vi "Real Time Display.vi"() -> ()   [LabVIEW 2015]
uses:
  Type/_Run Mode.ctl
  InternalTools/IonicsServiceTool/Print.ctl
  Type/_Data Operation.ctl
  Type/_RT Command.ctl
  Configuration/_Global Configuration.vi
  <vilib>/Utility/config.llb/Read Key (String).vi
  <vilib>/Utility/config.llb/Read Key (Double).vi
  <vilib>/Utility/config.llb/Read Key (I32).vi
  <vilib>/Utility/NIReport.llb/Append Image to Report (path wrap).vi
  <vilib>/Utility/NIReport.llb/NI_report.lvclass
  <vilib>/Utility/config.llb/NI_LVConfig.lvlib
panel:
  out "Close":bool
  out "Quit":bool=TRUE
  out "Q2DC POL":bool
  out "Q1DC POL":bool
  out "Date":string
  out "MCA":bool
  out "Run Mode":T1
  out "Q2 Resolution":i32[](listbox) caption="Q2 +ve High Res"
  out "Q1 Resolution":i32[](listbox) caption="Q1 +ve High Res"
  out "Q2 Calibration":i32[](listbox)
  out "Q1 Calibration":i32[](listbox)
  out "Scan #":i32=1
  out "Peak List":i32[](listbox)
  out "Lens Values":i32[](listbox)
  out "TIC":cluster{"TIC X":dbl[], "TIC Y":dbl[]}[](graph)
  out "Run Time":i32=1 caption="Run Time (ms)"
  in  "Expt#":i32=1 caption="Experiment #"
  out "Init":bool
  out "A 6":bool
  out "A 5":bool
  out "A 4":bool
  out "A 3":bool
  out "A 2":bool
  out "A 1":bool
  out "MR 5":cluster{dbl[], dbl[]}(graph)
  out "MR 4":cluster{dbl[], dbl[]}(graph)
  out "MR 2":cluster{dbl[], dbl[]}(graph)
  out "MR 1":cluster{dbl[], dbl[]}(graph)
  out "MR 6":cluster{dbl[], dbl[]}(graph)
  out "MR 3":cluster{dbl[], dbl[]}(graph)
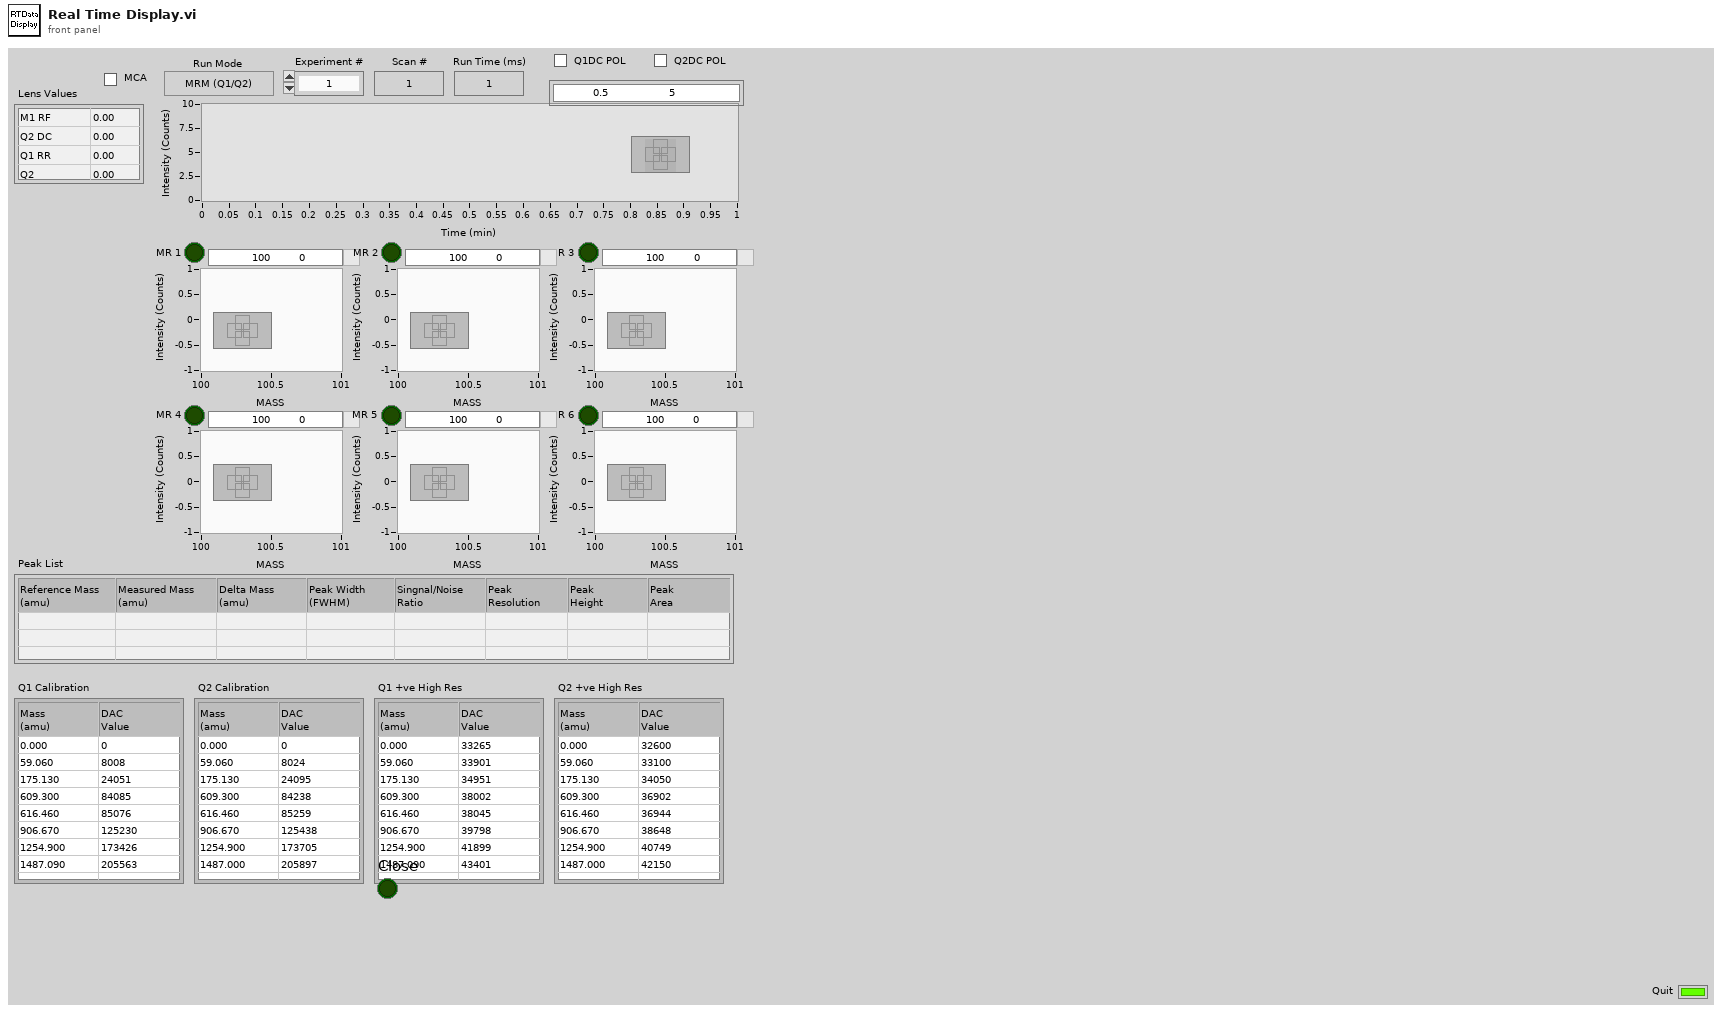
[diagram p1: front panel]
types:
  T1 = typedef "_Run Mode.ctl" = enum16{"MRM (Q1/Q2)", "Q1 Scan", "Q1 SRM", "Q2 Scan", "Q2 SRM", "Product Scan", "Precursor Scan", "Neutral Loss", "Neutral Gain"}
  T2 = cluster{"TIC":refnum<vi>, "MR 1":refnum<vi>, "MR 2":refnum<vi>, "MR 3":refnum<vi>, "MR 4":refnum<vi>, "MR 5":refnum<vi>, "MR 6":refnum<vi>, "A 1":refnum<vi>, "A 2":refnum<vi>, "A 3":refnum<vi>, "A 4":refnum<vi>, "A 5":refnum<vi>, "A 6":refnum<vi>, "Lens Values":refnum<vi>, "Q1 Calibration":refnum<vi>, "Q2 Calibration":refnum<vi>, "Q1 Resolution":refnum<vi>, "Q2 Resolution":refnum<vi>, "Peak List":refnum<vi>}
  T3 = cluster{"RefMass":dbl[], "LensList":i32[], "SearchWin":dbl, "MinH":dbl, "MinW":i32, "RunTime":i32}
  T4 = typedef "Print.ctl" = cluster{"Picture Name":string, "VI Reference":refnum<vi>}
  T5 = enum16{"Standard Report", "HTML", "Word", "Excel"}
  T6 = typedef "_Data Operation.ctl" = enum8{"Initialize", "Get Data", "Set Data", "Close"}
  T7 = typedef "_RT Command.ctl" = enum16{"xml Start Run", "xml Start Actual Run", "xml Stop Run", "xml Runtime Update", "xml Get Status", "xml Get Table", "xml Set Table", "xml Get Configuration", "xml System Status", "xml Set LC Input Logic", "xml Get Data", "xml Get Info", "Start", "StartActualRun", "Stop", "Runtime Update", "Get Data", "Get Info", "Get Status", "Get Param", "Get Config", "Get Table", "Read ADC", "Set Oscillator", "Update Config", "Update Table", "Set All Pol", "Set Pol and DC", "Set Max Mass", "Toggle RP", "Toggle EL", "Set PIC", "Initialize Turbo", "Send Turbo Comm", "Close Turbo", "P1", "P2", "P3", "Send Serial", "Set LC Out", "Get LC In", "Read VAC", "Test Table", "Toggle Power", "Get Startup", "Set Startup", "Get ADC Table", "Set ADC Table", "Get Brief Status", "Get Detail Status", "Auxiliary Update", "Set CC Logics", "Set CC Input Logics", "Ignore Error", "invalid"}
  T8 = typedef "NI_LVConfig.lvlib/Config Data RefNum.ctl" = refnum<k1>
  T9 = typedef "_Current Data.ctl" = cluster{"Scan#":i32, "Run Time (mS)":i32, "TIC X":dbl[], "TIC Y":dbl[][], "MassRange":cluster{"X Title":string, "X":dbl[], "Y":i32[]}[], "Fixed Mass (amu)":dbl, "Method":T10}
  T10 = typedef "_XML Expt.ctl" = cluster{"StartT(mS)":i32, "#Cycles":i32, "PauseT(uS)":i32, "ScanType":i32, "Polarity":u8, "FixedMass":dbl, "DelayT(mS)":i32, "Active Ch":T11[], "Mass Range":T12[]}
  T11 = typedef "_XML Lens.ctl" = cluster{"Value":dbl, "ChID":u8}
  T12 = typedef "_Mass Range Property.ctl" = cluster{"Start":dbl, "Stop":dbl, "Step Size":dbl, "Steps":i32, "Dwell":dbl, "Parameters":T13[], "Res":T14}
  T13 = typedef "_Mass Range Parameters.ctl" = cluster{"Name":string, "Ch#":u8, "StartV":dbl, "StopV":dbl, "StepV":dbl, "Index":u8}
  T14 = typedef "_RT Res Type.ctl" = u16
  T15 = typedef "_Peak Property.ctl" = cluster{"Centroid":dbl, "Height":dbl, "FWHM":dbl, "Resolution":dbl, "Area":dbl, "StoN":dbl, "ApexX":dbl, "Baseline":dbl, "LEdgeX":dbl, "LEdgeY":dbl, "REdgeX":dbl, "REdgeY":dbl, "LEdgeFWHM":dbl, "REdgeFWHM":dbl}
  T16 = typedef "imagedata.ctl" = cluster{"image type":i32, "image depth":i32, "image":u8[], "mask":u8[], "colors":u32[], "Rectangle":cluster{"left":i16, "top":i16, "right":i16, "bottom":i16}}
  T17 = typedef "LVRangeTypeDef.ctl" = cluster{"Minimum":dbl, "Maximum":dbl, "Increment":dbl, "Minor Increment":dbl, "Start":dbl}
  T18 = typedef "LVPointDoubleTypeDef.ctl" = cluster{"Cursor X":dbl, "Cursor Y":dbl}
  T19 = cluster{"YScale.NameLbl.Text":string, "XScale.NameLbl.Text":string, "XScale.Range":T17, "YScale.Range":T17, "Label.Text":string, "Cursor.Cursor Position":T18, "Plot.Bar Plot Style":u8}
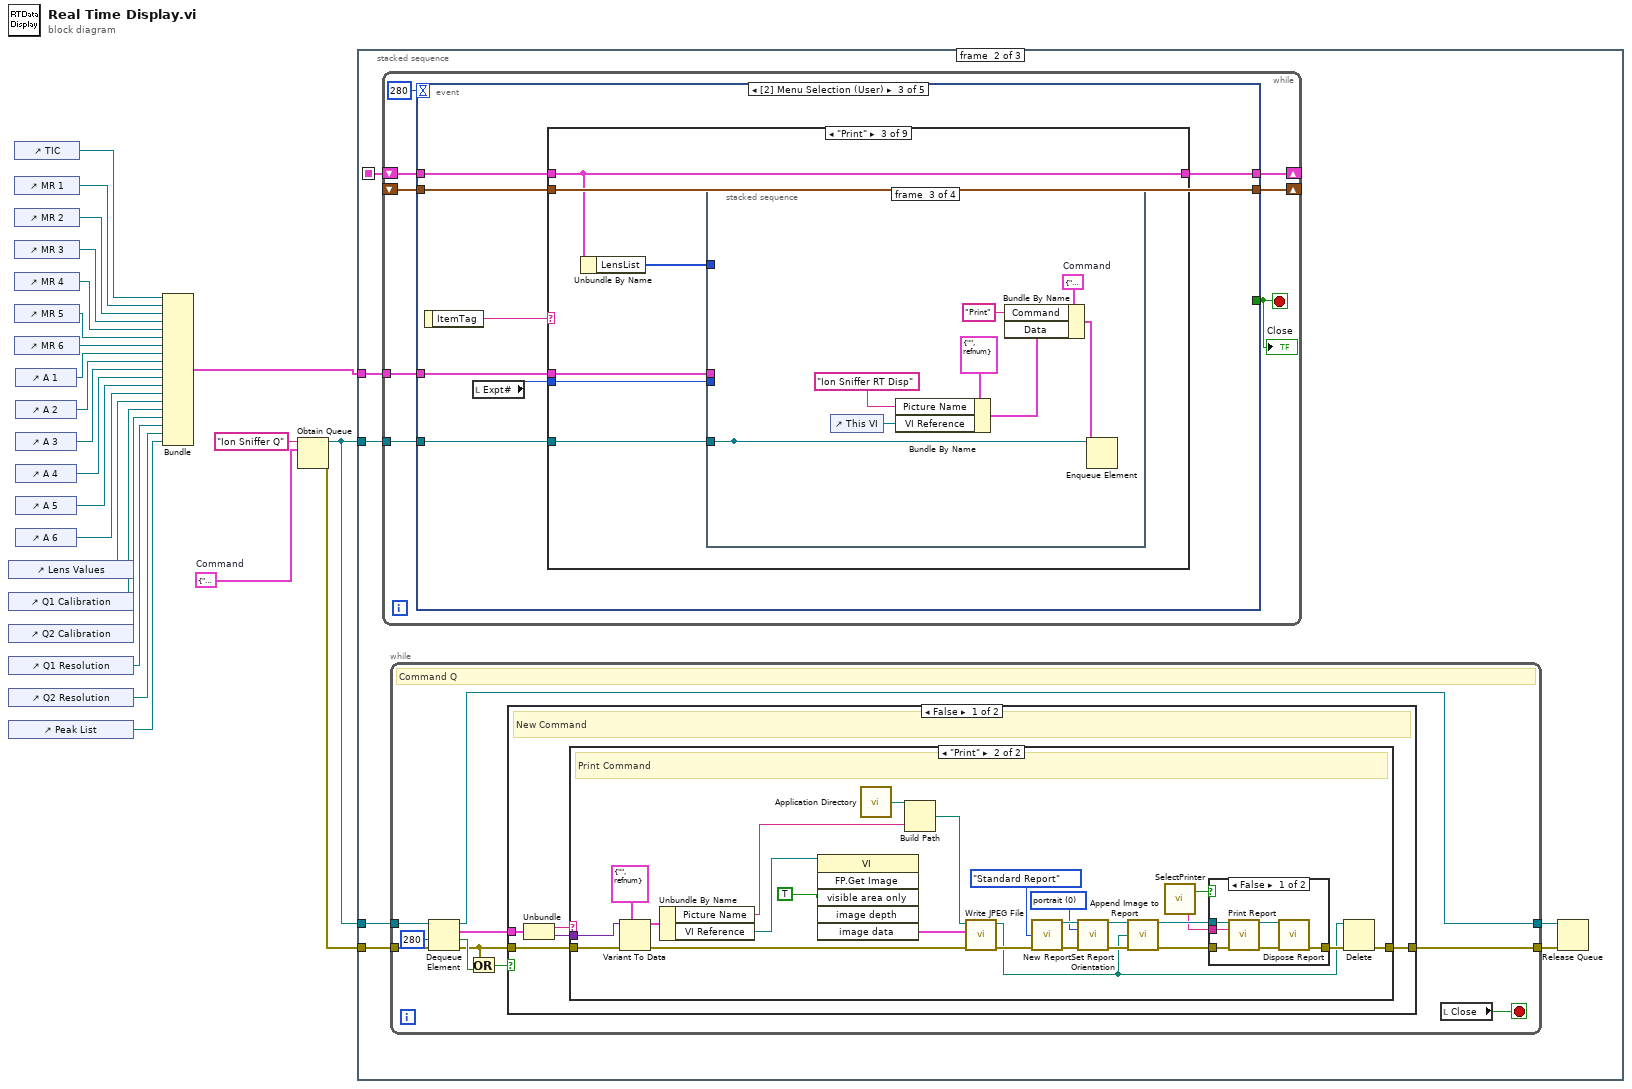
[diagram p0: block diagram]
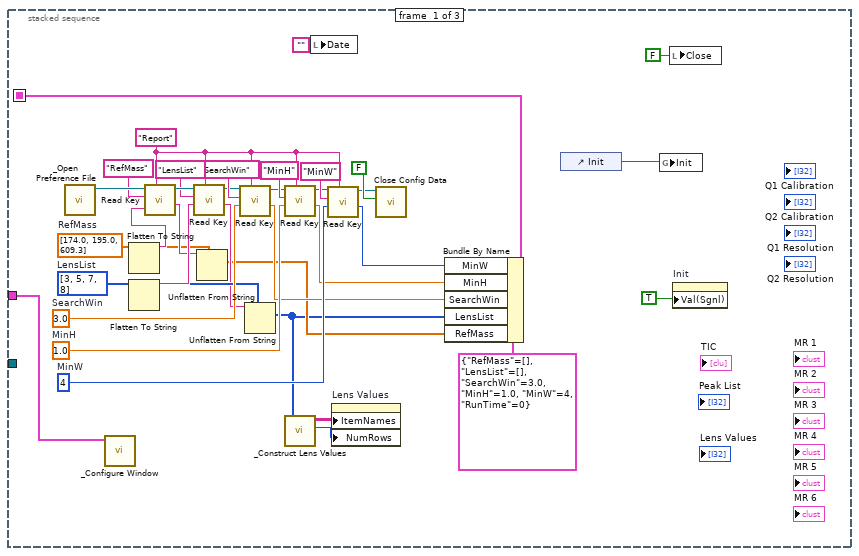
[diagram p2: hidden frame]
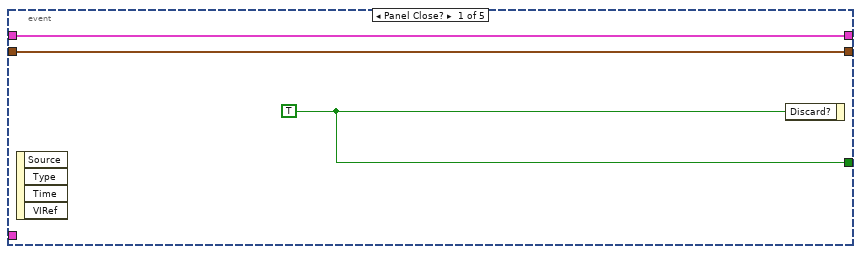
[diagram p6: hidden frame]
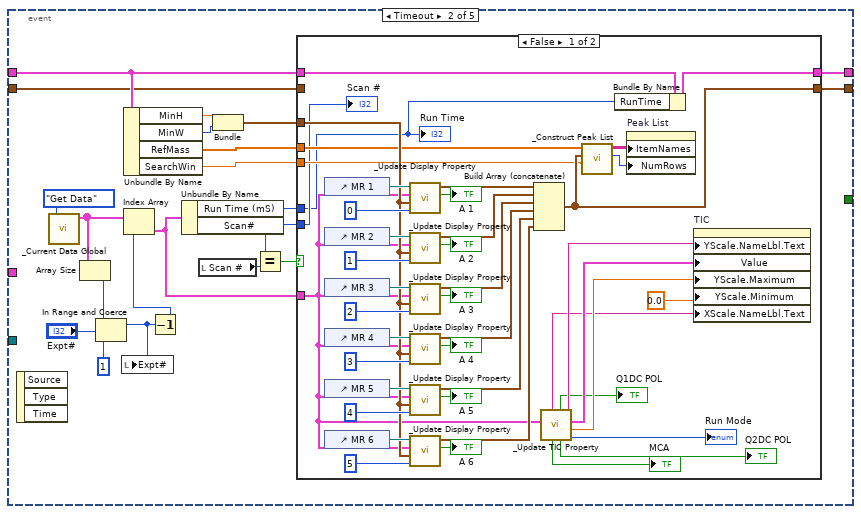
[diagram p7: hidden frame]
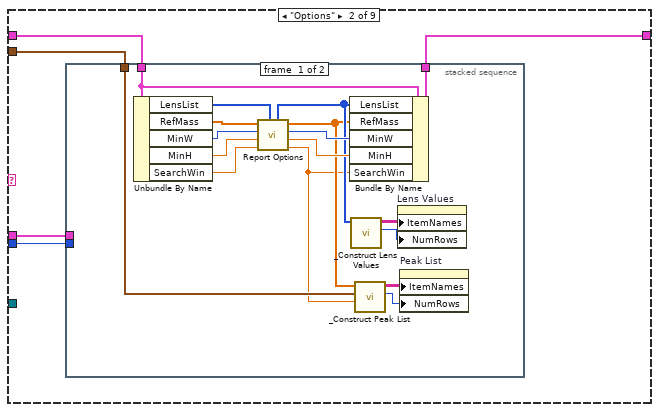
[diagram p10: hidden frame]
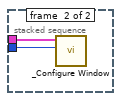
[diagram p11: hidden frame]
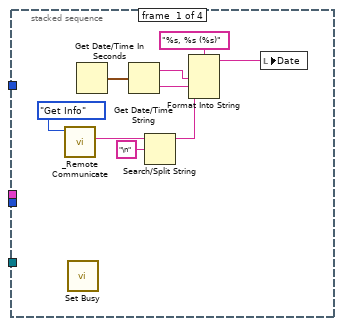
[diagram p12: hidden frame]
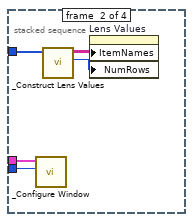
[diagram p13: hidden frame]
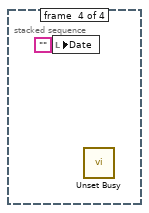
[diagram p14: hidden frame]
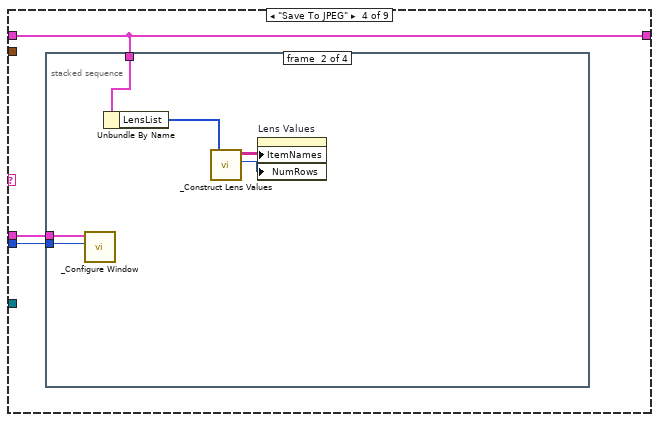
[diagram p15: hidden frame]
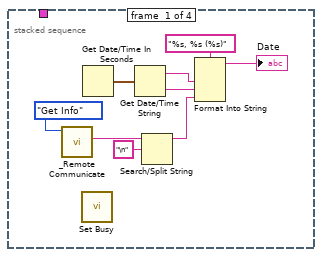
[diagram p16: hidden frame]
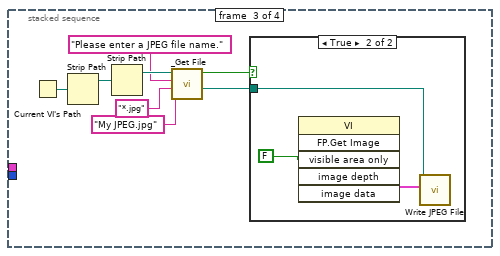
[diagram p17: hidden frame]
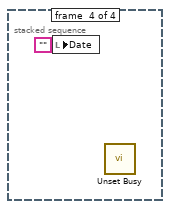
[diagram p19: hidden frame]
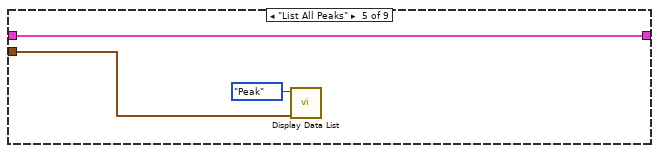
[diagram p20: hidden frame]
diagram:
  w1 = cluster{"Command":string, "Data":variant} {"Command"="", "Data"=variant}  # Command
  n1 = control-ref of="Lens Values"() -> (w24:refnum<vi>)
  n2 = control-ref of="Q1 Calibration"() -> (w10:refnum<vi>)
  n3 = control-ref of="Q2 Calibration"() -> (w9:refnum<vi>)
  n4 = control-ref of="Q1 Resolution"() -> (w8:refnum<vi>)
  n5 = control-ref of="Q2 Resolution"() -> (w7:refnum<vi>)
  n6 = control-ref of="Peak List"() -> (w6:refnum<vi>)
  n7 = control-ref of="TIC"() -> (w5:refnum<vi>)
  n8 = control-ref of="MR 1"() -> (w12:refnum<vi>)
  n9 = control-ref of="MR 2"() -> (w13:refnum<vi>)
  n10 = control-ref of="MR 3"() -> (w14:refnum<vi>)
  n11 = control-ref of="MR 4"() -> (w15:refnum<vi>)
  n12 = control-ref of="MR 5"() -> (w16:refnum<vi>)
  n13 = control-ref of="MR 6"() -> (w17:refnum<vi>)
  n14 = control-ref of="A 1"() -> (w18:refnum<vi>)
  n15 = control-ref of="A 2"() -> (w19:refnum<vi>)
  n16 = control-ref of="A 3"() -> (w20:refnum<vi>)
  n17 = control-ref of="A 4"() -> (w21:refnum<vi>)
  n18 = control-ref of="A 5"() -> (w22:refnum<vi>)
  n19 = control-ref of="A 6"() -> (w23:refnum<vi>)
  n20 = Bundle("TIC"=w5, "MR 1"=w12, "MR 2"=w13, "MR 3"=w14, "MR 4"=w15, "MR 5"=w16, "MR 6"=w17, "A 1"=w18, "A 2"=w19, "A 3"=w20, "A 4"=w21, "A 5"=w22, "A 6"=w23, "Lens Values"=w24, "Q1 Calibration"=w10, "Q2 Calibration"=w9, "Q1 Resolution"=w8, "Q2 Resolution"=w7, "Peak List"=w6) -> (w11:T2)  [unwired: 1 out]
  n21 = Obtain Queue(name (unnamed)="Ion Sniffer Q", element data type=w1) -> (queue out=w3:refnum<queue>, error out=w2:errorcluster)  [unwired: 3 in, 1 out]
  n22 = stacked-sequence {
    seq-local: [w31 _ _] -> [_ w67 _]
    tunnel: w11 -> [w27 w66 _]
    tunnel: w3 -> [_ w65 _]
    tunnel: w3 -> [_ w64 _]
    tunnel: w2 -> [_ w63 _]
    frame #0 {
      w47 = "Report" ("section")
      w38 = i32[] [3, 5, 7, 8]  # LensList
      w43 = 4  # MinW
      w44 = 1.0  # MinH
      w45 = 3.0  # SearchWin
      w39 = dbl[] [174.0, 195.0, 609.3]  # RefMass
      n23 = call "_Open Preference File.vi"() -> ("refnum"=w56:T8)  [unwired: 3 in, 4 out]
      n24 = call "_Configure Window.vi"("ControlRef"=w27) -> ()  [unwired: 2 in, 5 out]
      n25 = Flatten To String(anything=w39) -> (data string=w42:string)  [unwired: 1 in, 4 out]
      n26 = Flatten To String(anything=w38) -> (data string=w41:string)  [unwired: 1 in, 4 out]
      n27 = call-poly <vilib>:"Read Key.vi"("section"=w47, "default value"=w42, "key"="RefMass", "refnum"=w56) -> ("value"=w40:string, "refnum out"=w58:T8)  [unwired: 2 in, 4 out]
      n28 = call-poly <vilib>:"Read Key.vi"("section"=w47, "default value"=w41, "key"="LensList" ("section"), "refnum"=w58) -> ("value"=w37:string, "refnum out"=w50:T8)  [unwired: 2 in, 4 out]
      n29 = Unflatten From String(type=w39, binary string=w40) -> (value=w32:dbl[])  [unwired: 1 in, 4 out]
      n30 = call-poly <vilib>:"Read Key.vi"("section"=w47, "default value"=w45, "key"="SearchWin", "refnum"=w50) -> ("value"=w33:dbl, "refnum out"=w51:T8)  [unwired: 1 in, 5 out]
      n31 = Unflatten From String(type=w38, binary string=w37) -> (value=w30:i32[])  [unwired: 1 in, 4 out]
      n32 = call-poly <vilib>:"Read Key.vi"("section"=w47, "default value"=w44, "key"="MinH" ("section"), "refnum"=w51) -> ("value"=w34:dbl, "refnum out"=w48:T8)  [unwired: 1 in, 5 out]
      n33 = call "_Construct Lens Values.vi"("Lens List"=w30) -> ("# of Lens"=w28:i32, "Table"=w29:string[][])  [unwired: 5 out]
      n34 = local write "Date"("") -> ()
      n35 = call-poly <vilib>:"Read Key.vi"("section"=w47, "default value"=w43, "key"="MinW" ("section"), "refnum"=w48) -> ("value"=w35:i32, "refnum out"=w46:T8)  [unwired: 1 in, 5 out]
      n36 = property on="Lens Values" class="MCListbox (strict)"("ItemNames"=w29, "NumRows"=w28) -> ()  [unwired: 2 in, 2 out]
      n37 = call <vilib>:"Close Config Data.vi"("write file if changed (T)"=FALSE ("write configuration file? (F)"), "refnum"=w46) -> ()  [unwired: 1 in, 9 out]
      n38 = Bundle By Name(cluster=T3 {"RefMass"=[], "LensList"=[], "SearchWin"=3.0, "MinH"=1.0, "MinW"=4, "RunTime"=0}, "MinW"=w35, "MinH"=w34, "SearchWin"=w33, "LensList"=w30, "RefMass"=w32) -> (w31:T3)
      n39 = control-ref of="Init"() -> (w60:refnum<vi>)
      n40 = global write "_Global Configuration.vi" "Init"(w60) -> ()
      n41 = local write "Close"(FALSE ("Close")) -> ()
      n42 = property on="Init" class="Bool (strict)"("Val(Sgnl)"=TRUE ("Value (Signaling)")) -> ()  [unwired: 2 in, 2 out]
    }
    frame #1 {
      n43 = while {
        shift-right: [w123] -> _
        shift-left: w67 -> [w124]
        shift-right: [w122] -> _
        shift-left: _ -> [w121]
        tunnel: w66 -> [w120]
        tunnel: w65 -> [w118]
        stop <- w117 stop-if-true
        n44 = event shown="[2] Menu Selection (User)" {
          selector: _ -> [_ _ _ _ _]
          dyn-events: _ -> [_ _ _ _ _]
          timeout: 280 -> [_ _ _ _ _]
          tunnel: [w127 _ _ _ _] -> w117
          tunnel: w124 -> [w126 w148 w200 w312 w318]
          tunnel: [w126 w147 w199 w313 w318] -> w123
          tunnel: [w125 w145 w198 w308 w317] -> w122
          tunnel: w121 -> [w125 w146 w198 w308 w317]
          tunnel: w120 -> [_ _ w197 w306 _]
          tunnel: w118 -> [_ _ w195 _ _]
          event Panel Close? {
            w127 = TRUE ("Discard?")
            n45 = event-data() -> ()  [unwired: 5 out]
            n46 = event-data("Discard?"=w127) -> ()  [unwired: 1 in, 1 out]
          }
          event Timeout {
            n47 = event-data() -> ()  [unwired: 4 out]
            n48 = call "_Current Data Global.vi"("Operation"=_Data_Operation."Get Data") -> ("CurrentData"=w137:T9[])  [unwired: 3 in, 3 out]
            n49 = Array Size(array=w137) -> (size(s)=w134:i32)
            n50 = In Range and Coerce(upper limit=w134, x="Expt#", lower limit=1) -> (coerced(x)=w133:i32)  [unwired: 1 out]
            n51 = local write "Expt#"(w133) -> ()
            n52 = Unbundle By Name(w148) -> ("MinH"=w143:dbl, "MinW"=w142:i32, "RefMass"=w140:dbl[], "SearchWin"=w139:dbl)
            n53 = Decrement(x=w133) -> (x-1=w132:i32)
            n54 = Index Array(array=w137, index=w132) -> (element=w138:T9)
            n55 = Unbundle By Name(w138) -> ("Run Time (mS)"=w128:i32, "Scan#"=w130:i32)
            n56 = local read "Scan #"() -> (w131:i32)
            n57 = Bundle("MinH"=w143, "MinW"=w142) -> (w141:cluster{"MinH":dbl, "MinW":i32})  [unwired: 1 out]
            n58 = Equal?(x=w130, y=w131) -> (x = y?=w129:bool)
            n59 = case shown="False" w129 {
              tunnel: w148 -> [w192 w194]
              tunnel: [w191 w194] -> w147
              tunnel: [w163 w193] -> w145
              tunnel: w146 -> [_ w193]
              tunnel: w141 -> [w177 _]
              tunnel: w138 -> [w159 _]
              tunnel: w140 -> [w162 _]
              tunnel: w139 -> [w161 _]
              tunnel: w130 -> [w160 _]
              tunnel: w128 -> [w152 _]
              frame False {
                n60 = control-ref of="MR 1"() -> (w190:refnum<vi>)
                n61 = control-ref of="MR 2"() -> (w189:refnum<vi>)
                n62 = control-ref of="MR 3"() -> (w187:refnum<vi>)
                n63 = control-ref of="MR 4"() -> (w185:refnum<vi>)
                n64 = control-ref of="MR 5"() -> (w183:refnum<vi>)
                n65 = control-ref of="MR 6"() -> (w181:refnum<vi>)
                n66 = call "_Update Display Property.vi"("MassRange# (0)"=0, "PeakParam"=w177, "Current Data"=w159, "Display Refnum"=w190) -> ("Active"=→"A 1":bool, "Peak List"=w171:T15[])  [unwired: 3 out]
                n67 = call "_Update Display Property.vi"("MassRange# (0)"=1, "PeakParam"=w177, "Current Data"=w159, "Display Refnum"=w189) -> ("Active"=→"A 2":bool, "Peak List"=w170:T15[])  [unwired: 3 out]
                n68 = call "_Update Display Property.vi"("MassRange# (0)"=2, "PeakParam"=w177, "Current Data"=w159, "Display Refnum"=w187) -> ("Active"=→"A 3":bool, "Peak List"=w169:T15[])  [unwired: 3 out]
                n69 = call "_Update Display Property.vi"("MassRange# (0)"=3, "PeakParam"=w177, "Current Data"=w159, "Display Refnum"=w185) -> ("Active"=→"A 4":bool, "Peak List"=w168:T15[])  [unwired: 3 out]
                n70 = call "_Update Display Property.vi"("MassRange# (0)"=4, "PeakParam"=w177, "Current Data"=w159, "Display Refnum"=w183) -> ("Active"=→"A 5":bool, "Peak List"=w167:T15[])  [unwired: 3 out]
                n71 = call "_Update Display Property.vi"("MassRange# (0)"=5, "PeakParam"=w177, "Current Data"=w159, "Display Refnum"=w181) -> ("Active"=→"A 6":bool, "Peak List"=w166:T15[])  [unwired: 3 out]
                n72 = Build Array (concatenate)(w171, w170, w169, w168, w167, w166) -> (w163:T15[])
                n73 = call "_Update TIC Property.vi"("Current Data"=w159) -> ("Run Mode"=→"Run Mode":T1, "YMax"=w156:dbl, "TIC Data"=w157:cluster{"TIC X":dbl[], "Data in cps":dbl[]}[], "YTitle"=w158:string, "Q2DC Pol"=→"Q2DC POL":bool, "Q1DC Pol"=→"Q1DC POL":bool, "MCA"=→"MCA":bool, "XTitle"=w151:string)  [unwired: 3 out]
                n74 = call "_Construct Peak List.vi"("Search Window"=w161, "Peak List"=w163, "RefMass"=w162) -> ("# of Peaks"=w164:i32, "Table"=w165:string[][])  [unwired: 3 out]
                n75 = Bundle By Name(cluster=w192, "RunTime"=w152) -> (w191:T3)
                n76 = property on="Peak List" class="MCListbox (strict)"("ItemNames"=w165, "NumRows"=w164) -> ()  [unwired: 2 in, 2 out]
                n77 = property on="TIC" class="XYGraph (strict)"("YScale.NameLbl.Text"=w158, "Value"=w157, "YScale.Maximum"=w156, "YScale.Minimum"=0.0 ("Y Scale.Range:Minimum"), "XScale.NameLbl.Text"=w151) -> ()  [unwired: 2 in, 2 out]
                "Run Time" <- w152
                "Scan #" <- w160
              }
              frame True {
              }
            }
          }
          event Menu Selection (User) {
            n78 = event-data() -> ("ItemTag"=w201:string)  [unwired: 1 out]
            n79 = local read "Expt#"() -> (w196:i32)
            n80 = case shown="\"Print\"" w201 {
              tunnel: w200 -> [w202 w207 w231 w257 w287 w288 w291 w293 w305]
              tunnel: [w202 w206 w231 w257 w287 w288 w291 w293 w305] -> w199
              tunnel: w198 -> [_ w205 _ _ w286 _ _ _ _]
              tunnel: w197 -> [_ w204 w229 w256 _ _ _ w294 w304]
              tunnel: w196 -> [_ w203 w228 w255 _ _ _ w292 w303]
              tunnel: w195 -> [_ _ w227 _ _ _ _ _ _]
              frame Default {
              }
              frame "Options" {
                n81 = stacked-sequence {
                  tunnel: w207 -> [w208 _]
                  tunnel: [w219 _] -> w206
                  tunnel: w205 -> [w216 _]
                  tunnel: w204 -> [_ w226]
                  tunnel: w203 -> [_ w225]
                  frame #0 {
                    n82 = Unbundle By Name(w208) -> ("LensList"=w224:i32[], "RefMass"=w215:dbl[], "MinW"=w223:i32, "MinH"=w222:dbl, "SearchWin"=w214:dbl)
                    n83 = call "Report Options.vi"("LensList"=w224, "Search Window"=w214, "Min. Height"=w222, "Min. Width"=w223, "RefMass"=w215) -> ("Search Window 2"=w209:dbl, "Min. Height 2"=w220:dbl, "Min. Width 2"=w221:i32, "RefMass 2"=w210:dbl[], "LensList 2"=w211:i32[])
                    n84 = Bundle By Name(cluster=w208, "LensList"=w211, "RefMass"=w210, "MinW"=w221, "MinH"=w220, "SearchWin"=w209) -> (w219:T3)
                    n85 = call "_Construct Lens Values.vi"("Lens List"=w211) -> ("# of Lens"=w212:i32, "Table"=w213:string[][])  [unwired: 5 out]
                    n86 = call "_Construct Peak List.vi"("Search Window"=w209, "Peak List"=w216, "RefMass"=w210) -> ("# of Peaks"=w217:i32, "Table"=w218:string[][])  [unwired: 3 out]
                    n87 = property on="Lens Values" class="MCListbox (strict)"("ItemNames"=w213, "NumRows"=w212) -> ()  [unwired: 2 in, 2 out]
                    n88 = property on="Peak List" class="MCListbox (strict)"("ItemNames"=w218, "NumRows"=w217) -> ()  [unwired: 2 in, 2 out]
                  }
                  frame #1 {
                    n89 = call "_Configure Window.vi"("Expt#"=w225, "ControlRef"=w226) -> ()  [unwired: 1 in, 5 out]
                  }
                }
              }
              frame "Print" {
                n90 = Unbundle By Name(w231) -> ("LensList"=w230:i32[])
                n91 = stacked-sequence {
                  tunnel: w230 -> [_ w243 _ _]
                  tunnel: w229 -> [_ w242 _ _]
                  tunnel: w228 -> [_ w241 _ _]
                  tunnel: [_ _ w253 _] -> _
                  tunnel: w227 -> [_ _ w253 _]
                  frame #0 {
                    n92 = call "_Remote Communicate.vi"("Command"=_RT_Command."Get Info") -> ("Info"=w239:string)  [unwired: 5 in, 3 out]
                    n93 = call <vilib>:"Set Busy.vi"() -> ()  [unwired: 4 in, 8 out]
                    n94 = Get Date/Time In Seconds() -> (seconds since 1Jan1904=w237:timestamp)
                    n95 = Get Date/Time String(seconds (now)=w237) -> (date string=w235:string, time string=w234:string)  [unwired: 2 out]
                    n96 = Search/Split String(string=w239, search string/char (-)="\n") -> (substring before match=w233:string)  [unwired: 3 out]
                    n97 = Format Into String(format string="%s, %s (%s)", w235, w234, w233) -> (resulting string=w232:string)  [unwired: 2 in, 1 out]
                    n98 = local write "Date"(w232) -> ()
                  }
                  frame #1 {
                    n99 = call "_Configure Window.vi"("Expt#"=w241, "ControlRef"=w242) -> ()  [unwired: 1 in, 5 out]
                    n100 = call "_Construct Lens Values.vi"("Lens List"=w243) -> ("# of Lens"=w244:i32, "Table"=w245:string[][])  [unwired: 5 out]
                    n101 = property on="Lens Values" class="MCListbox (strict)"("ItemNames"=w245, "NumRows"=w244) -> ()  [unwired: 2 in, 2 out]
                  }
                  frame #2 {
                    w252 = cluster{"Command":string, "Data":variant} {"Command"="", "Data"=variant}  # Command
                    n102 = control-ref of="This VI"() -> (w247:refnum<vi>)
                    n103 = Bundle By Name(cluster=T4 {"Picture Name"="", "VI Reference"=refnum} ("Cluster"), "Picture Name"="Ion Sniffer RT Disp", "VI Reference"=w247) -> (w246:T4)
                    n104 = Bundle By Name(cluster=w252, "Command"="Print", "Data"=w246) -> (w250:cluster{"Command":string, "Data":variant})
                    n105 = Enqueue Element(queue=w253, element=w250) -> ()  [unwired: 2 in, 3 out]
                  }
                  frame #3 {
                    n106 = local write "Date"("") -> ()
                    n107 = call <vilib>:"Unset Busy.vi"() -> ()  [unwired: 2 in, 10 out]
                  }
                }
              }
              frame "Save To JPEG" {
                n108 = stacked-sequence {
                  tunnel: w257 -> [_ w270 _ _]
                  tunnel: w256 -> [_ w268 _ _]
                  tunnel: w255 -> [_ w267 _ _]
                  frame #0 {
                    n109 = call "_Remote Communicate.vi"("Command"=_RT_Command."Get Info") -> ("Info"=w265:string)  [unwired: 5 in, 3 out]
                    n110 = call <vilib>:"Set Busy.vi"() -> ()  [unwired: 4 in, 8 out]
                    n111 = Get Date/Time In Seconds() -> (seconds since 1Jan1904=w263:timestamp)
                    n112 = Get Date/Time String(seconds (now)=w263) -> (date string=w261:string, time string=w260:string)  [unwired: 2 out]
                    n113 = Search/Split String(string=w265, search string/char (-)="\n") -> (substring before match=w259:string)  [unwired: 3 out]
                    n114 = Format Into String(format string="%s, %s (%s)", w261, w260, w259) -> (resulting string=→"Date":string)  [unwired: 2 in, 1 out]
                  }
                  frame #1 {
                    n115 = call "_Configure Window.vi"("Expt#"=w267, "ControlRef"=w268) -> ()  [unwired: 1 in, 5 out]
                    n116 = Unbundle By Name(w270) -> ("LensList"=w269:i32[])
                    n117 = call "_Construct Lens Values.vi"("Lens List"=w269) -> ("# of Lens"=w271:i32, "Table"=w272:string[][])  [unwired: 5 out]
                    n118 = property on="Lens Values" class="MCListbox (strict)"("ItemNames"=w272, "NumRows"=w271) -> ()  [unwired: 2 in, 2 out]
                  }
                  frame #2 {
                    n119 = Current VI's Path() -> (path=w280:path)
                    n120 = Strip Path(path=w280) -> (stripped path=w279:path)  [unwired: 1 out]
                    n121 = Strip Path(path=w279) -> (stripped path=w278:path)  [unwired: 1 out]
                    n122 = call "_Get File.vi"("default name"="My JPEG.jpg", "extension (isd)"="*.jpg", "prompt"="Please enter a JPEG file name.", "Start Path"=w278) -> ("Seleted File"=w274:path, "Succeeded"=w275:bool)  [unwired: 2 in, 2 out]
                    n123 = case shown="True" w275 {
                      tunnel: w274 -> [_ w281]
                      frame False {
                      }
                      frame True {
                        n124 = invoke class="VI" method="FP.Get Image"("visible area only"=FALSE ("Visible Area Only")) -> ("image data"=w282:T16)  [unwired: 5 in, 5 out]
                        n125 = call <vilib>:"Write JPEG File.vi"("image data"=w282, "path to JPEG file"=w281) -> ()  [unwired: 1 in, 9 out]
                      }
                    }
                  }
                  frame #3 {
                    n126 = local write "Date"("") -> ()
                    n127 = call <vilib>:"Unset Busy.vi"() -> ()  [unwired: 2 in, 10 out]
                  }
                }
              }
              frame "List All Peaks" {
                n128 = call "Display Data List.vi"("Peak List"=w286, "Data Type"=enum16{"TIC", "Spectrum", "Peak"}."Peak") -> ()  [unwired: 8 out]
              }
              frame "List TIC Data" {
                n129 = call "Display Data List.vi"("Data Type"=enum16{"TIC", "Spectrum", "Peak"}."TIC") -> ()  [unwired: 3 in, 6 out]
              }
              frame "List Spectral Data" {
                n130 = call "Display Data List.vi"("Data Type"=enum16{"TIC", "Spectrum", "Peak"}."Spectrum") -> ()  [unwired: 1 in, 8 out]
              }
              frame "Show Lens Values" {
                n131 = flat-sequence {
                  tunnel: w294 -> [w296]
                  tunnel: w292 -> [w295]
                  tunnel: w293 -> [w298]
                  frame #0 {
                    n132 = call "_Configure Window.vi"("For Printing (T)"=TRUE ("For Printing (F)"), "Expt#"=w295, "ControlRef"=w296) -> ()  [unwired: 5 out]
                  }
                  frame #1 {
                    n133 = Unbundle By Name(w298) -> ("LensList"=w299:i32[])
                    n134 = call "_Construct Lens Values.vi"("Lens List"=w299) -> ("# of Lens"=w300:i32, "Table"=w301:string[][])  [unwired: 5 out]
                    n135 = property on="Lens Values" class="MCListbox (strict)"("ItemNames"=w301, "NumRows"=w300) -> ()  [unwired: 2 in, 2 out]
                  }
                }
              }
              frame "Hide Lens Values" {
                n136 = call "_Configure Window.vi"("For Printing (T)"=FALSE, "Expt#"=w303, "ControlRef"=w304) -> ()  [unwired: 5 out]
              }
            }
          }
          event "Init": Value Change {
            w307 = 0 ("RunTime")
            # "This event must be sent at the start of each run"
            n137 = event-data() -> ()  [unwired: 7 out]
            n138 = Unbundle By Name(w312) -> ("LensList"=w309:i32[])
            n139 = call "_Configure Window.vi"("ControlRef"=w306) -> ()  [unwired: 2 in, 5 out]
            n140 = call "_Construct Lens Values.vi"("Lens List"=w309) -> ("# of Lens"=w310:i32, "Table"=w311:string[][])  [unwired: 5 out]
            n141 = property on="Lens Values" class="MCListbox (strict)"("ItemNames"=w311, "NumRows"=w310) -> ()  [unwired: 2 in, 2 out]
            n142 = Bundle By Name(cluster=w312, "RunTime"=w307) -> (w313:T3)
            n143 = local write "Scan #"(w307) -> ()
            n144 = local write "Run Time"(w307) -> ()
            "Init" <- FALSE ("Init")
          }
          event "MR 1", "MR 2", "MR 3", "MR 4", "MR 5", "MR 6", "TIC": Mouse Down? {
            n145 = event-data() -> ("CtlRef"=w315:refnum<vi>, "Mods.Double Click"=w316:bool)  [unwired: 4 out]
            n146 = case shown="True" w316 {
              tunnel: w315 -> [_ w333]
              frame False {
              }
              frame True {
                n147 = call "_Launch Dynamic VI.vi"("VI Name"=path "Show One Plot.vi" ("name or relative path")) -> ("VI Refnum"=w335:refnum<vi>)  [unwired: 3 out]
                n148 = property class="XYGraph"(reference=w333) -> ("YScale.NameLbl.Text"=w331:string, "XScale.NameLbl.Text"=w330:string, "XScale.Range"=w329:T17, "YScale.Range"=w328:T17, "Label.Text"=w327:string, "Cursor.Cursor Position"=w326:T18, "Plot.Bar Plot Style"=w319:u8)  [unwired: 1 in, 2 out]
                n149 = property class="VI"(reference=w335) -> (reference out=w338:refnum<vi>, error out=w337:errorcluster, "Front Panel"=w336:refnum<vi>)  [unwired: 1 in]
                n150 = property class="Pnl"(reference=w336, error in=w337) -> (error out=w324:errorcluster, "Controls[]"=w325:refnum<vi>[])  [unwired: 1 out]
                n151 = Bundle("YScale.NameLbl.Text"=w331, "XScale.NameLbl.Text"=w330, "XScale.Range"=w329, "YScale.Range"=w328, "Label.Text"=w327, "Cursor.Cursor Position"=w326, "Plot.Bar Plot Style"=w319) -> (w321:T19)  [unwired: 1 out]
                n152 = To Variant(anything=w321) -> (Variant=w320:variant)
                n153 = call "_Get Server Control.vi"("error in (no error)"=w324, "Control Name"="Data", "All Controls[]"=w325) -> ("error out"=w332:errorcluster, "Ctl Refnum"=w322:refnum<vi>)  [unwired: 3 out]
                n154 = property class="Ctl"(reference=w322, "Val(Sgnl)"=w320) -> ()  [unwired: 1 in, 2 out]
                n155 = Close Reference(reference=w338, error in (no error)=w332) -> ()  [unwired: 1 out]
              }
            }
            n156 = event-data() -> ()  [unwired: 1 in, 5 out]
          }
        }
        "Close" <- w117
      }
      n157 = while {
        tunnel: w64 -> [w76]
        tunnel: w63 -> [w77]
        tunnel: [w73] -> w61
        tunnel: [w72] -> w62
        stop <- w68 stop-if-true
        # "Command Q"
        n158 = Dequeue Element(queue=w76, timeout in ms (-1)=280, error in (no error)=w77) -> (queue out=w72:refnum<queue>, element=w75:cluster{"Command":string, "Data":variant}, timed out?=w71:bool, error out=w70:errorcluster)
        n159 = Or(x=w70, y=w71) -> (x .or. y?=w69:bool)
        n160 = case shown="False" w69 {
          tunnel: w70 -> [w79 w116]
          tunnel: w75 -> [w82 _]
          tunnel: [w78 w116] -> w73
          frame False {
            # "New Command"
            n161 = Unbundle(w82) -> ("Command"=w80:string, "Data"=w81:variant)
            n162 = case shown="\"Print\"" w80 {
              tunnel: w81 -> [_ w84]
              tunnel: w79 -> [w83 w106]
              tunnel: [w83 w91] -> w78
              frame Default {
                # "unknown command"
              }
              frame "Print" {
                w96 = 0 items=["portrait", "landscape"] ("orientation (portrait)")
                # "Print Command"
                n163 = Variant To Data(error in=w106, type=T4 {"Picture Name"="", "VI Reference"=refnum} ("Cluster"), Variant=w84) -> (data=w87:T4, error out=w89:errorcluster)
                n164 = Unbundle By Name(w87) -> ("Picture Name"=w86:string, "VI Reference"=w85:refnum<vi>)
                n165 = invoke class="VI" method="FP.Get Image"(reference=w85, "visible area only"=TRUE ("Visible Area Only")) -> ("image data"=w107:T16)  [unwired: 4 in, 5 out]
                n166 = call <vilib>:"Application Directory.vi"() -> ("Application Directory"=w105:path)
                n167 = Build Path(base path=w105, name or relative path=w86) -> (appended path=w104:path)
                n168 = call <vilib>:"Write JPEG File.vi"("error in (no error)"=w89, "image data"=w107, "path to JPEG file"=w104) -> ("error out"=w93:errorcluster, "path"=w90:path)  [unwired: 7 out]
                n169 = call <vilib>:"New Report.vi"("report type"=T5."Standard Report", "error in (no error)"=w93) -> ("report out"=w97:refnum<class "NI_report.lvclass">, "error out"=w101:errorcluster)  [unwired: 12 in]
                n170 = call-dynamic "Set Report Orientation.vi"("report in"=w97, "orientation (portrait)"=w96, "error in (no error)"=w101) -> ("report out"=w99:refnum<class "NI_report.lvclass">, "error out"=w102:errorcluster)  [unwired: 11 in]
                n171 = call-poly <vilib>:"Append Image to Report.vi"("report in"=w99, "path or URL of image"=w90, "error in (no error)"=w102) -> ("report out"=w100:refnum<class "NI_report.lvclass">, "error out"=w103:errorcluster)  [unwired: 9 in, 2 out]
                n172 = call "SelectPrinter.vi"() -> ("ChosenPrinter"=w95:string, "Closed?"=w94:bool)  [unwired: 2 in]
                n173 = case shown="False" w94 {
                  tunnel: w100 -> [w114 _]
                  tunnel: w95 -> [w112 _]
                  tunnel: w103 -> [w111 w115]
                  tunnel: [w109 w115] -> w92
                  frame False {
                    n174 = call-dynamic "Print Report.vi"("report in"=w114, "printer name (default)"=w112, "error in (no error)"=w111) -> ("report out"=w113:refnum<class "NI_report.lvclass">, "error out"=w110:errorcluster)  [unwired: 11 in]
                    n175 = call-dynamic "Dispose Report.vi"("report in"=w113, "error in (no error)"=w110) -> ("error out"=w109:errorcluster)  [unwired: 13 in]
                  }
                  frame True {
                  }
                }
                n176 = Delete(path (use dialog)=w90, error in=w92) -> (error out=w91:errorcluster)  [unwired: 3 in, 2 out]
              }
            }
          }
          frame True {
            # "Timeout/Error"
          }
        }
        n177 = local read "Close"() -> (w68:bool)
      }
      n178 = Release Queue(queue=w62, error in (no error)=w61) -> ()  [unwired: 1 in, 3 out]
    }
    frame #2 {
      n179 = property class="VI"("Front Panel.Open"=FALSE ("Front Panel Window:Open")) -> ()  [unwired: 2 in, 2 out]
    }
  }
